vi "niRFUtil CAL Band Data to Table.vi"(9 "Calibration Data":T1 {"Calibration Table" min=0 max=127 format="%.2p"; "Time Stamp (sec)" format="%^.2e"; "Temperature (C)" format="%.1f"}) -> (1 "Table (frequency, power, pathloss)":sgl[][](array[numeric]))   [LabVIEW 2015, in "niRFUtil.lvlib"]
uses:
  niRFUtil.lvlib
  Includes/niRFUtil INC Calibration Data.ctl
  Includes/niRFUtil INC Calibration Table.ctl
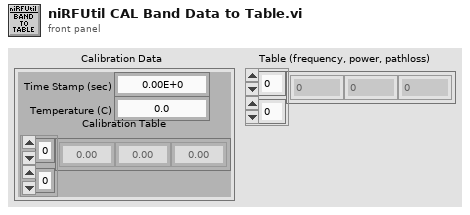
[diagram p1: front panel]
types:
  T1 = typedef "niRFUtil.lvlib/niRFUtil INC Calibration Data.ctl" = cluster{"Temperature (C)":dbl, "Time Stamp (sec)":dbl, "Calibration Table":T2}
  T2 = typedef "niRFUtil.lvlib/niRFUtil INC Calibration Table.ctl" = sgl[][]
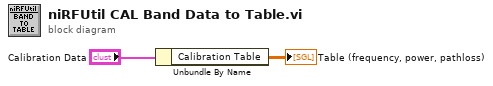
[diagram p0: block diagram]
diagram:
  n1 = Unbundle By Name("Calibration Data") -> ("Calibration Table"=→"Table (frequency, power, pathloss)":T2)
